vi "Populate Body Text Data.vi"(10 "Text settings":T2 {"Alignment" items=["left", "center", "right"]}, 11 "Text":T1) -> (3 "Body Text":T5 {"Body Text Spec"."Alignment" items=["left", "center", "right"]})   [LabVIEW 2020, in "LabVIEW Icon API.lvlib"]
doc: "Transform the Body Text data into a new cluster."
uses:
  LabVIEW Icon API.lvlib
  lv_icon/Controls/Alignment.ctl
  lv_icon/Controls/Font.ctl
  lv_icon/Controls/BodyText.ctl
  API_Text Colors.ctl
  API_Test Settings.ctl
  API_Text.ctl
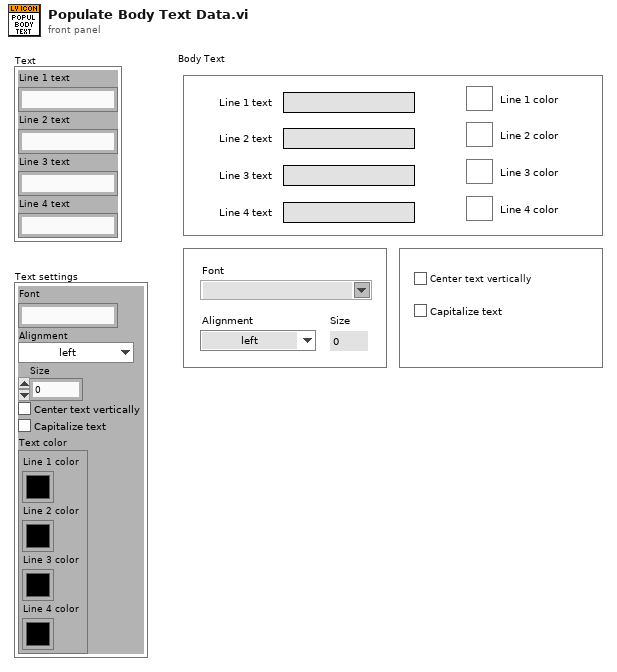
[diagram p1: front panel]
types:
  T1 = typedef "LabVIEW Icon API.lvlib/API_Text.ctl" = cluster{"Line 1 text":string, "Line 2 text":string, "Line 3 text":string, "Line 4 text":string}
  T2 = typedef "LabVIEW Icon API.lvlib/API_Test Settings.ctl" = cluster{"Font":string, "Alignment":T3, "Size":u8, "Center text":bool, "Capitalize text":bool, "Text color":T4}
  T3 = typedef "Alignment.ctl" = u16
  T4 = typedef "LabVIEW Icon API.lvlib/API_Text Colors.ctl" = cluster{"Line 1 color":u32, "Line 2 color":u32, "Line 3 color":u32, "Line 4 color":u32}
  T5 = typedef "BodyText.ctl" = cluster{"Line 1 text":string, "Line 2 text":string, "Line 3 text":string, "Line 4 text":string, "Line 1 color":u32, "Line 2 color":u32, "Line 3 color":u32, "Line 4 color":u32, "Body Text Spec":cluster{"Font":T6, "Alignment":T3, "Size":u8}, "Center text vertically":bool, "Capitalize Text":bool}
  T6 = typedef "Font.ctl" = string
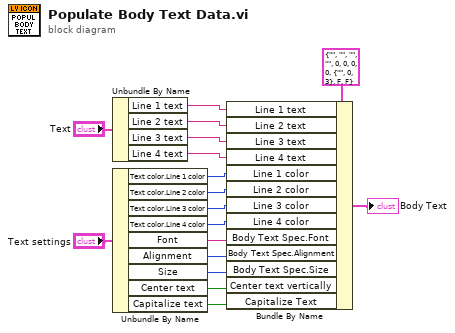
[diagram p0: block diagram]
diagram:
  n1 = Unbundle By Name("Text") -> ("Line 1 text"=w3:string, "Line 2 text"=w6:string, "Line 3 text"=w5:string, "Line 4 text"=w4:string)
  n2 = Unbundle By Name("Text settings") -> ("Text color.Line 1 color"=w8:u32, "Text color.Line 2 color"=w9:u32, "Text color.Line 3 color"=w10:u32, "Text color.Line 4 color"=w11:u32, "Font"=w12:string, "Alignment"=w13:T3, "Size"=w14:u8, "Center text"=w15:bool, "Capitalize text"=w16:bool)
  n3 = Bundle By Name(cluster=T5 {"Line 1 text"="", "Line 2 text"="", "Line 3 text"="", "Line 4 text"="", "Line 1 color"=0, "Line 2 color"=0, "Line 3 color"=0, "Line 4 color"=0, "Body Text Spec"={"Font"="", "Alignment"=0, "Size"=3}, "Center text vertically"=FALSE, "Capitalize Text"=FALSE} ("Body Text"), "Line 1 text"=w3, "Line 2 text"=w6, "Line 3 text"=w5, "Line 4 text"=w4, "Line 1 color"=w8, "Line 2 color"=w9, "Line 3 color"=w10, "Line 4 color"=w11, "Body Text Spec.Font"=w12, "Body Text Spec.Alignment"=w13, "Body Text Spec.Size"=w14, "Center text vertically"=w15, "Capitalize Text"=w16) -> (→"Body Text":T5)
